vi "oa_Angular Speed Calculation.vi"(6 "deltaX":dbl format="%.2f", 7 "reset? (True)":bool=TRUE, 8 "pulse future [s]":dbl[](array[numeric]) format="%.2f", 9 "pulse history in  [s]":dbl[](array[numeric]) format="%.2f", 10 "pulse new history in  [s]":dbl[](array[numeric]) format="%.2f", 11 "pulse positions in [s]":dbl[](array[numeric]) format="%.2f") -> (0 "dY/dX[n]":dbl[](array[numeric]) format="%.2f", 1 "pulse history out  [s]":dbl[](array[numeric]) format="%.2f", 2 "pulse new history out  [s]":dbl[](array[numeric]) format="%.2f", 3 "pulse positions out [s]":dbl[](array[numeric]) format="%.2f")   [LabVIEW 2017, in "SoundVib_TachProcess.lvlib"]
uses:
  <vilib>/addons/Sound and Vibration/Order Analysis/Tach Process/SoundVib_TachProcess.lvlib
  <vilib>/Analysis/2dsp.llb/1D Convolution (DBL).vi
  <vilib>/Analysis/NI_AALPro.lvlib
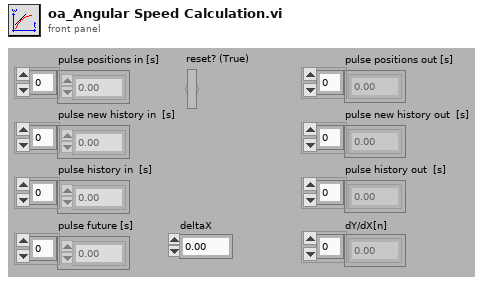
[diagram p1: front panel]
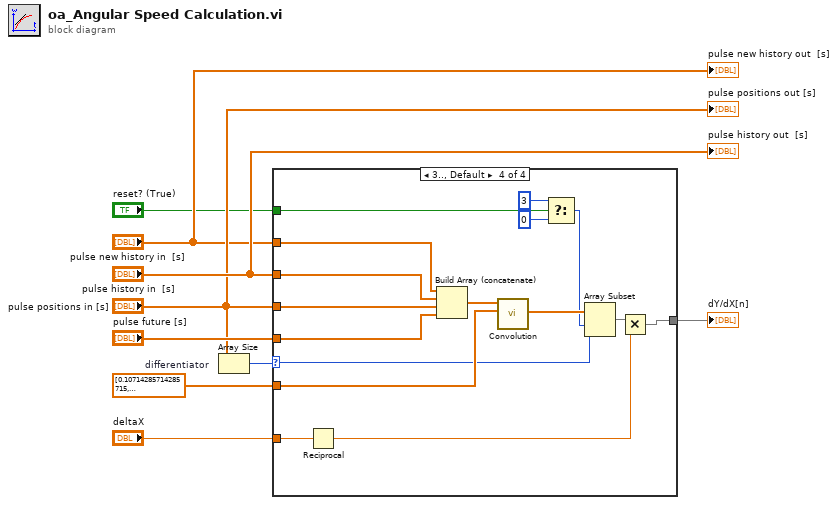
[diagram p0: block diagram]
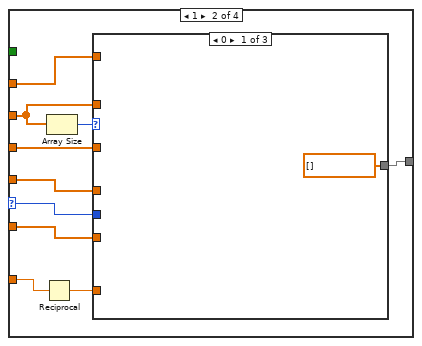
[diagram p3: hidden frame]
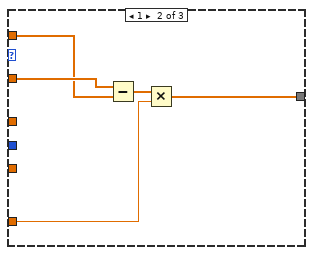
[diagram p4: hidden frame]
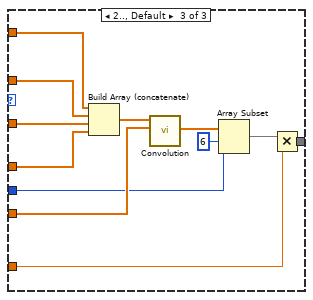
[diagram p5: hidden frame]
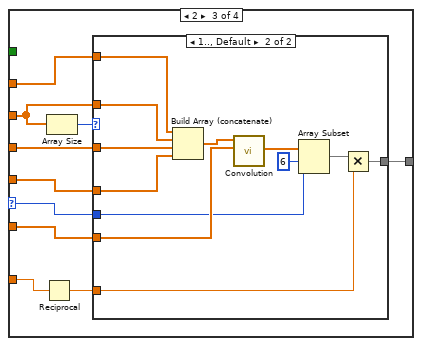
[diagram p6: hidden frame]
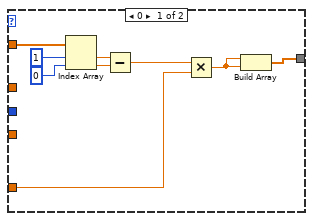
[diagram p7: hidden frame]
diagram:
  w7 = dbl[] [0.10714285714285715, 0.07142857142857142, 0.035714285714285705, -1.5209319782164736e-17, -0.03571428571428571, -0.07142857142857142, -0.10714285714285715]  # differentiator
  n1 = Array Size(array="pulse positions in [s]") -> (size(s)=w3:i32)
  n2 = case shown="3.., Default" w3 {
    selector: w3 -> [_ w15 w43 w80]
    tunnel: [_ w19 w47 w84] -> w9
    tunnel: "deltaX" -> [_ w12 w40 w78]
    tunnel: w7 -> [_ w18 w46 w83]
    tunnel: "pulse future [s]" -> [_ w17 w45 w82]
    tunnel: "pulse history in  [s]" -> [_ w13 w41 w79]
    tunnel: "pulse positions in [s]" -> [_ w16 w44 w81]
    tunnel: "pulse new history in  [s]" -> [_ w10 w38 w73]
    tunnel: "reset? (True)" -> [_ _ _ w72]
    frame 0 {
    }
    frame 1 {
      n3 = Reciprocal(x=w12) -> (1/x=w11:dbl)
      n4 = Array Size(array=w13) -> (size(s)=w14:i32)
      n5 = case shown="0" w14 {
        tunnel: [dbl[] [] w21 w35] -> w19
        tunnel: w11 -> [_ w22 w27]
        tunnel: w18 -> [_ _ w33]
        tunnel: w17 -> [_ _ w32]
        tunnel: w13 -> [_ w24 w31]
        tunnel: w16 -> [_ w25 w30]
        tunnel: w15 -> [_ _ w29]
        tunnel: w10 -> [_ _ w26]
        frame 0 {
        }
        frame 1 {
          n6 = Subtract(x=w25, y=w24) -> (x-y=w23:dbl[])
          n7 = Multiply(x=w23, y=w22) -> (x*y=w21:dbl[])
        }
        frame 2.., Default {
          n8 = Build Array (concatenate)(w26, w31, w30, w32) -> (w28:dbl[])
          n9 = call-poly <vilib>:"Convolution.vi"("Y"=w33, "X"=w28) -> ("X * Y"=w36:dbl[])  [unwired: 8 in, 1 out]
          n10 = Array Subset(array=w36, index=6, length=w29) -> (w37:dbl[])
          n11 = Multiply(x=w37, y=w27) -> (x*y=w35:dbl[])
        }
      }
    }
    frame 2 {
      n12 = Reciprocal(x=w40) -> (1/x=w39:dbl)
      n13 = Array Size(array=w41) -> (size(s)=w42:i32)
      n14 = case shown="1.., Default" w42 {
        tunnel: [w48 w66] -> w47
        tunnel: w39 -> [w50 w58]
        tunnel: w46 -> [_ w64]
        tunnel: w45 -> [_ w63]
        tunnel: w41 -> [_ w62]
        tunnel: w44 -> [w56 w61]
        tunnel: w43 -> [_ w60]
        tunnel: w38 -> [_ w57]
        frame 0 {
          n15 = Index Array(array=w56, index #1=1 ("index"), index #2=0 ("index")) -> (element #1=w53:dbl, element #2=w52:dbl)
          n16 = Subtract(x=w53, y=w52) -> (x-y=w51:dbl)
          n17 = Multiply(x=w51, y=w50) -> (x*y=w49:dbl)
          n18 = Build Array(w49, w49) -> (w48:dbl[])
        }
        frame 1.., Default {
          n19 = Build Array (concatenate)(w57, w62, w61, w63) -> (w59:dbl[])
          n20 = call-poly <vilib>:"Convolution.vi"("Y"=w64, "X"=w59) -> ("X * Y"=w67:dbl[])  [unwired: 8 in, 1 out]
          n21 = Array Subset(array=w67, index=6, length=w60) -> (w68:dbl[])
          n22 = Multiply(x=w68, y=w58) -> (x*y=w66:dbl[])
        }
      }
    }
    frame 3.., Default {
      n23 = Reciprocal(x=w78) -> (1/x=w77:dbl)
      n24 = Build Array (concatenate)(w73, w79, w81, w82) -> (w74:dbl[])
      n25 = call-poly <vilib>:"Convolution.vi"("Y"=w83, "X"=w74) -> ("X * Y"=w75:dbl[])  [unwired: 8 in, 1 out]
      n26 = Select(t=3, s=w72, f=0) -> (s? t:f=w69:i32)
      n27 = Array Subset(array=w75, index=w69, length=w80) -> (w76:dbl[])
      n28 = Multiply(x=w76, y=w77) -> (x*y=w84:dbl[])
    }
  }
  "dY/dX[n]" <- w9
  "pulse positions out [s]" <- "pulse positions in [s]"
  "pulse history out  [s]" <- "pulse history in  [s]"
  "pulse new history out  [s]" <- "pulse new history in  [s]"
